vi "Clamp Until Held, Then Lift.vi"(1 "Iterations":i32=1, 2 "Clamp + Lift":bool) -> ()   [LabVIEW 2014]
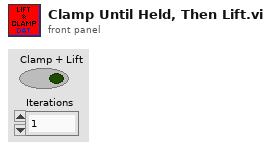
[diagram p1: front panel]
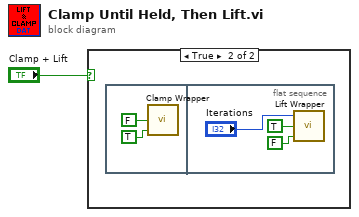
[diagram p0: block diagram]
diagram:
  n1 = case shown="True" "Clamp + Lift" {
    frame False {
    }
    frame True {
      n2 = flat-sequence {
        frame #0 {
          n3 = call "Clamp Wrapper.vi"("In"=TRUE ("In or Out"), "Out"=FALSE) -> ()  [unwired: 1 in]
        }
        frame #1 {
          n4 = call "Lift Wrapper.vi"("Down"=FALSE ("Up or Down"), "Up"=TRUE ("Up or Down"), "Iterations"="Iterations") -> ()
        }
      }
    }
  }
